vi "valve_VCH visu.vi"(10 "ALR":cluster{"ALRL1":bool, "ALRL2":bool}, 11 "Z":T3={"Z_Source"=1, "Z_SetState"=0, "Z_State"=0, "Z_State_T"=0, "ZM_State"=0, "ZM_State_T"=0, "ALR  L1"=FALSE, "ALR  L2"=FALSE, "HH_run"=0}) -> (2 "reset out":bool, 3 "Z_SetState":T1={"Z_HSw"=1, "Z_HSetState"=enum."initialization", "Reset_ALR"=FALSE}, 5 "This VI":refnum<vi>)   [LabVIEW 2019, in "Valves.lvlib"]
uses:
  Valves.lvlib
  ctl/Z_short.ctl
  ctl/Zr_control_VCH.ctl
  ctl/Z_State_VCH.ctl
  ctl/ZM_State_VCH.ctl
  Counter/Generator.vi
  Logik/fronts.vi
  Trigers/RS.vi
  Trigers/D^.vi
  Timer Delay/Timer.vi
  Timer Delay/Timers.lvlib
panel:
  in  "on":bool=TRUE
  in  "ALRL1_reset":bool
  in  "ALRL2_reset":bool
  in  "Z_HSwitch":bool=TRUE
  out "Z1 ind":u8(ring)
  out "Z3_ind":u16(ring)
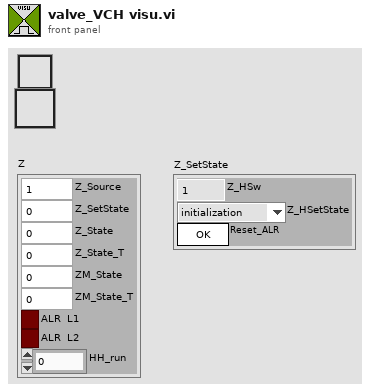
[diagram p1: front panel]
types:
  T1 = typedef "Valves.lvlib/Zr_control_VCH.ctl" = cluster{"Z_HSw":u8, "Z_HSetState":T2, "Reset_ALR":bool}
  T2 = typedef "Valves.lvlib/Z_State_VCH.ctl" = enum8{"initialization", "alarm", "disabled", "not ready", "closed ready", "reserv", "reserv1", "reserv2", "reserv3", "check", "on min", "open", "on (closed)"}
  T3 = typedef "Valves.lvlib/Z_short.ctl" = cluster{"Z_Source":u8, "Z_SetState":u8, "Z_State":u8, "Z_State_T":u32, "ZM_State":u8, "ZM_State_T":u32, "ALR  L1":bool, "ALR  L2":bool, "HH_run":i32}
  T4 = typedef "Valves.lvlib/ZM_State_VCH.ctl" = enum8{"initialization", "closed", "big_pause", "little_pause", "open", "close_cmd"}
  T5 = enum8{"Enabled", "Disabled", "Disabled and Grayed Out"}
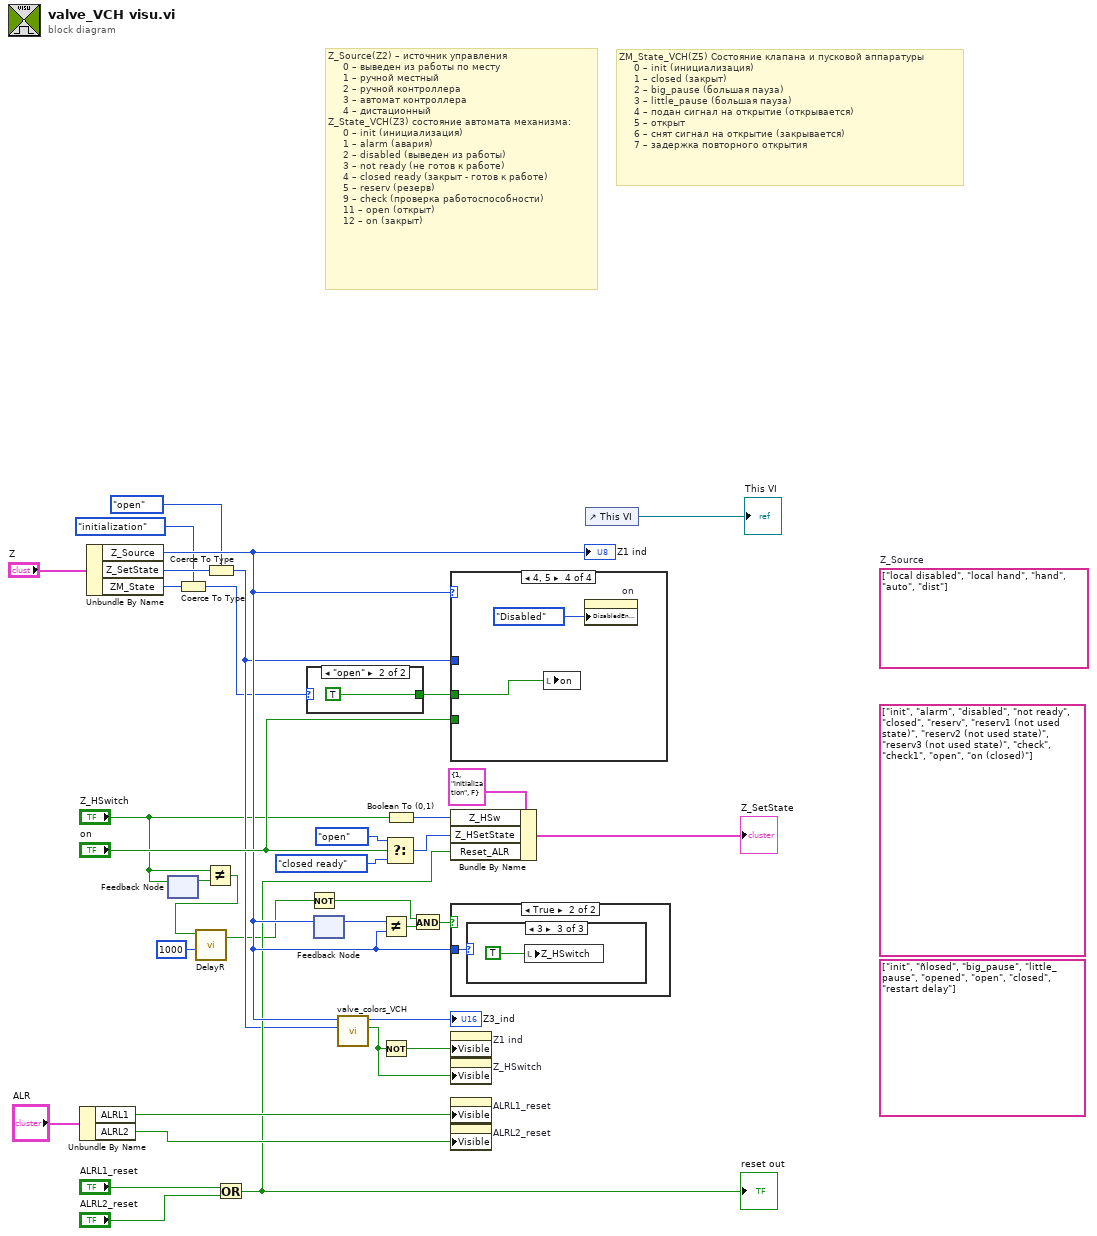
[diagram p0: block diagram]
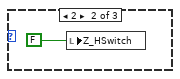
[diagram p5: hidden frame]
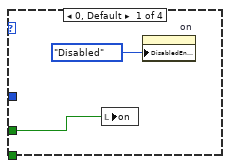
[diagram p6: hidden frame]
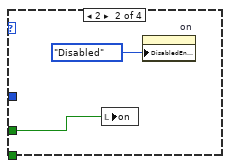
[diagram p7: hidden frame]
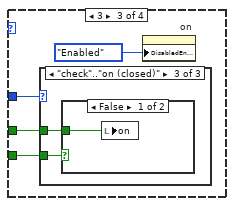
[diagram p8: hidden frame]
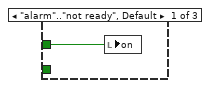
[diagram p9: hidden frame]
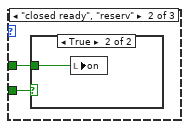
[diagram p10: hidden frame]
diagram:
  (unwired) string[] ["init", "alarm", "disabled", "not ready", "closed", "reserv", "reserv1 (not used state)", "reserv2 (not used state)", "reserv3 (not used state)", "check", "check1", "open", "on (closed)"]
  (unwired) string[] ["local disabled", "local hand", "hand", "auto", "dist"]  # Z_Source
  (unwired) string[] ["init", "ñlosed", "big_pause", "little_pause", "opened", "open", "closed", "restart delay"]
  # "Z_Source(Z2) – источник управления\n     0 – выведен из работы по месту\n     1 – ручной местный\n     2 – ручной контроллера\n     3 – автомат контроллера\n     4 – дистационный\nZ_State_VCH(Z3) состояние автомата механизма:\n     0 – init (инициализация)\n     1 – alarm (авария)\n     2 – disabled (выведен из работы)\n     3 – not ready (не готов к работе)\n     4 – closed ready (закрыт - готов к работе)\n     5 – reserv (резерв)\n     9 – check (проверка работоспособности)\n     11 – open (открыт)\n     12 – on (закрыт)"
  # "ZM_State_VCH(Z5) Состояние клапана и пусковой аппаратуры\n     0 – init (инициализация)\n     1 – сlosed (закрыт)\n     2 – big_pause (большая пауза)\n     3 – little_pause (большая пауза)\n     4 – подан сигнал на открытие (открывается)\n     5 – открыт\n     6 – снят сигнал на открытие (закрывается)\n     7 – задержка повторного открытия"
  n1 = Unbundle By Name("ALR") -> ("ALRL1"=w27:bool, "ALRL2"=w28:bool)
  n2 = Unbundle By Name("Z") -> ("Z_Source"=w26:u8, "Z_SetState"=w14:u8, "ZM_State"=w11:u8)
  "Z1 ind" <- w26
  n3 = feedback #1() -> (w8:bool)  [unwired: 1 in]
  n4 = feedback-in #1("Z_HSwitch") -> ()
  n5 = Coerce To Type(0:w11, 1:ZM_State_VCH."initialization" ("Z_State_VCH")) -> (2:w10:T4)
  n6 = Not Equal?(x="Z_HSwitch", y=w8) -> (x != y?=w6:bool)
  n7 = call "DelayR.vi"("DelayOff"=u32 1000, "In"=w6) -> ("Out"=w2:bool)  [unwired: 2 in, 1 out]
  n8 = Coerce To Type(0:w14, 1:Z_State_VCH."open" ("Z_HSetState")) -> (2:w12:T2)
  n9 = Or(x="ALRL1_reset", y="ALRL2_reset") -> (x .or. y?=w15:bool)
  "reset out" <- w15
  n10 = case shown="\"open\"" w10 {
    tunnel: [_ TRUE] -> w21
    frame "initialization", Default {
    }
    frame "open" {
    }
  }
  n11 = Not(x=w2) -> (.not. x?=w1:bool)
  n12 = feedback #2() -> (w30:u8)  [unwired: 1 in]
  n13 = feedback-in #2(w26) -> ()
  n14 = call "valve_colors_VCH.vi"("Z_State"=w12, "Z1(CmdSource)"=w26) -> ("auto visible"=w25:bool, "N ring"=→"Z3_ind":u16)  [unwired: 6 in, 2 out]
  n15 = Not Equal?(x=w30, y=w26) -> (x != y?=w3:bool)
  n16 = Not(x=w25) -> (.not. x?=w31:bool)
  n17 = Select(t=Z_State_VCH."open" ("Z_HSetState"), s="on", f=Z_State_VCH."closed ready" ("Z_HSetState")) -> (s? t:f=w33:T2)
  n18 = Boolean To (0,1)(Boolean="Z_HSwitch") -> (0, 1=w34:i16)
  n19 = And(x=w1, y=w3) -> (x .and. y?=w4:bool)
  n20 = case shown="4, 5" w26 {
    tunnel: w21 -> [w37 w39 w42 w52]
    tunnel: w12 -> [_ _ w43 _]
    tunnel: "on" -> [_ _ w41 _]
    frame 0, Default {
      n21 = local write "on"(w37) -> ()
      n22 = property on="on" class="Bool (strict)"("DisabledEnum"=T5."Disabled" ("Disabled")) -> ()  [unwired: 2 in, 2 out]
    }
    frame 2 {
      n23 = local write "on"(w39) -> ()
      n24 = property on="on" class="Bool (strict)"("DisabledEnum"=T5."Disabled" ("Disabled")) -> ()  [unwired: 2 in, 2 out]
    }
    frame 3 {
      n25 = case shown="\"check\"..\"on (closed)\"" w43 {
        tunnel: w42 -> [w45 w46 w49]
        tunnel: w41 -> [_ w47 w50]
        frame "alarm".."not ready", Default {
          n26 = local write "on"(w45) -> ()
        }
        frame "closed ready", "reserv" {
          n27 = case shown="True" w47 {
            tunnel: w46 -> [_ w48]
            frame False {
            }
            frame True {
              n28 = local write "on"(w48) -> ()
            }
          }
        }
        frame "check".."on (closed)" {
          n29 = case shown="False" w50 {
            tunnel: w49 -> [w51 _]
            frame False {
              n30 = local write "on"(w51) -> ()
            }
            frame True {
            }
          }
        }
      }
      n31 = property on="on" class="Bool (strict)"("DisabledEnum"=T5."Enabled" ("Disabled")) -> ()  [unwired: 2 in, 2 out]
    }
    frame 4, 5 {
      n32 = local write "on"(w52) -> ()
      n33 = property on="on" class="Bool (strict)"("DisabledEnum"=T5."Disabled" ("Disabled")) -> ()  [unwired: 2 in, 2 out]
    }
  }
  n34 = Bundle By Name(cluster=T1 {"Z_HSw"=1, "Z_HSetState"=enum."initialization", "Reset_ALR"=FALSE} ("Z_SetState 2"), "Z_HSw"=w34, "Z_HSetState"=w33, "Reset_ALR"=w15) -> (→"Z_SetState":T1)
  n35 = case shown="True" w4 {
    tunnel: w26 -> [_ w54]
    frame False {
    }
    frame True {
      n36 = case shown="3" w54 {
        frame 0, Default {
        }
        frame 2 {
          n37 = local write "Z_HSwitch"(FALSE ("Z_ASwitch")) -> ()
        }
        frame 3 {
          n38 = local write "Z_HSwitch"(TRUE ("Z_ASwitch")) -> ()
        }
      }
    }
  }
  n39 = property on="Z1 ind" class="Ring (strict)"("Visible"=w31) -> ()  [unwired: 2 in, 2 out]
  n40 = property on="Z_HSwitch" class="Bool (strict)"("Visible"=w25) -> ()  [unwired: 2 in, 2 out]
  n41 = property on="ALRL1_reset" class="Bool (strict)"("Visible"=w27) -> ()  [unwired: 2 in, 2 out]
  n42 = property on="ALRL2_reset" class="Bool (strict)"("Visible"=w28) -> ()  [unwired: 2 in, 2 out]
  n43 = control-ref of="This VI"() -> (→"This VI":refnum<vi>)
